vi "Current Output_Buffer_Dbl_VIG.vi"(6 "Automatic":bool=TRUE, 7 "Operation":T1(ring)=enum."set data", 8 "error in":errorcluster, 11 "Numeric":dbl) -> (0 "error out":errorcluster, 3 "Numeric":dbl)   [LabVIEW 2010]
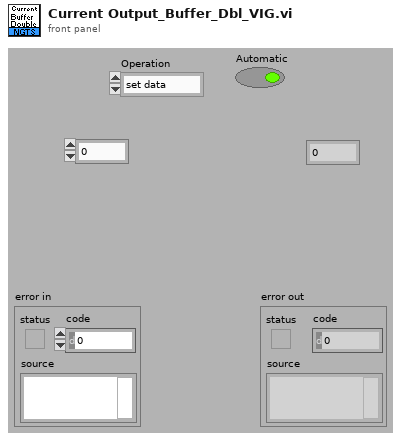
[diagram p1: front panel]
types:
  T1 = enum16{"get data", "set data", "Set Mode", "initialize"}
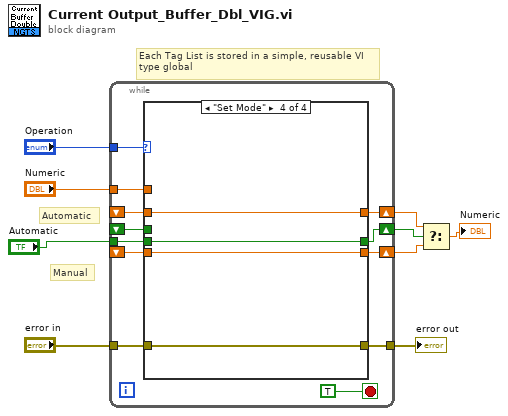
[diagram p0: block diagram]
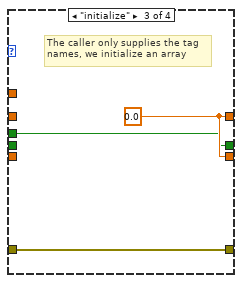
[diagram p5: hidden frame]
diagram:
  # "Automatic"
  # "Manual"
  # "Each Tag List is stored in a simple, reusable VI\ntype global"
  n1 = while {
    tunnel: "Operation" -> [w21]
    shift-right: [w19] -> w4
    shift-left: _ -> [w17]
    tunnel: "Numeric" -> [w18]
    tunnel: "error in" -> [w16]
    tunnel: [w15] -> w6
    shift-right: [w14] -> w3
    shift-left: _ -> [w13]
    shift-right: [w11] -> w1
    shift-left: _ -> [w12]
    tunnel: "Automatic" -> [w10]
    stop <- TRUE stop-if-true
    n2 = case shown="\"Set Mode\"" w21 {
      tunnel: [w25 w31 w38 w43] -> w19
      tunnel: w18 -> [_ w30 _ _]
      tunnel: w17 -> [w25 w27 _ w43]
      tunnel: w16 -> [w24 w32 w39 w40]
      tunnel: [w24 w32 w39 w40] -> w15
      tunnel: [w23 w29 w38 w42] -> w14
      tunnel: w13 -> [w23 w28 _ w42]
      tunnel: w12 -> [w22 w26 w37 _]
      tunnel: [w22 w26 w37 w41] -> w11
      tunnel: w10 -> [_ _ _ w41]
      frame "get data", Default {
      }
      frame "set data" {
        n3 = case shown="False" w26 {
          tunnel: [w33 w36] -> w31
          tunnel: w30 -> [w34 w36]
          tunnel: [w34 w35] -> w29
          tunnel: w28 -> [_ w35]
          tunnel: w27 -> [w33 _]
          frame False {
          }
          frame True {
          }
        }
      }
      frame "initialize" {
        w38 = 0.0 ("element")
        # "The caller only supplies the tag\nnames, we initialize an array"
      }
      frame "Set Mode" {
      }
    }
  }
  "error out" <- w6
  n4 = Select(t=w4, s=w1, f=w3) -> (s? t:f=→"Numeric":dbl)
